vi "tsapp_configure_can_regs.vi"(8 "错误输入（无错误）":errorcluster, 10 "Cluster":T1, 11 "path":path) -> (0 "错误输出":errorcluster, 2 "Return Type":i32, 3 "path out":path)   [LabVIEW 2014]
doc: "Function Introduction :\nConfigure CAN sampling points and baud rate\nCall location :\nAfter connecting the hardware, it is necessary to create a diagnostic module\ninput parameter :\nAIdxChn: Channel Index\nABaud rate Kbps: baud rate\nASEG1: Arbitration Stage Phase Buffer Stage 1 ASEG2: Arbitration Stage Phase Buffer Stage 2 APrescaler: Arbitration Stage Frequency Division Coefficient\nASJW: BTL quantity\nAOnlyListen: Is it in listen only mode\nA120OhmConnected: Is the 120 Ω terminal resistor activated\nReturn value :\n0: Execution successful\nOther values: Failed"
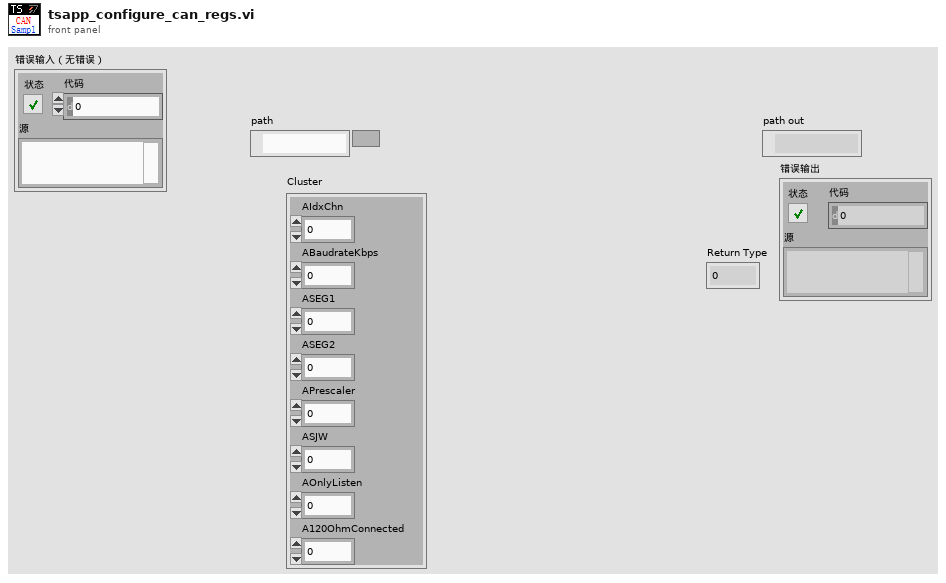
[diagram p1: front panel]
types:
  T1 = cluster{"AIdxChn":i32, "ABaudrateKbps":sgl, "ASEG1":i32, "ASEG2":i32, "APrescaler":i32, "ASJW":i32, "AOnlyListen":i32, "A120OhmConnected":i32}
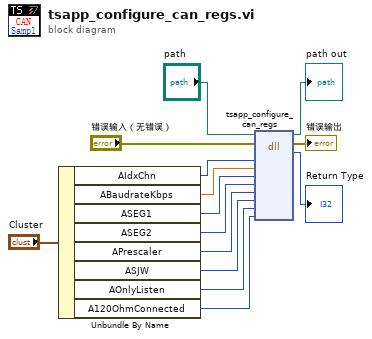
[diagram p0: block diagram]
diagram:
  n1 = Unbundle By Name("Cluster") -> ("AIdxChn"=w11:i32, "ABaudrateKbps"=w10:sgl, "ASEG1"=w8:i32, "ASEG2"=w9:i32, "APrescaler"=w7:i32, "ASJW"=w6:i32, "AOnlyListen"=w3:i32, "A120OhmConnected"=w4:i32)
  n2 = dll-call lib="C:/Users/XYY/Desktop/LabView Demo/TSCAN_LB2018_V1.3_20220301/Config/TSMaster.dll" fn="tsapp_configure_can_regs"(path in="path", error in="错误输入（无错误）", "AIdxChn"=w11, "ABaudrateKbps"=w10, "ASEG1"=w8, "ASEG2"=w9, "APrescaler"=w7, "ASJW"=w6, "AOnlyListen"=w3, "A120OhmConnected"=w4) -> (path out=→"path out":path, error out=→"错误输出":errorcluster, "返回类型"=→"Return Type":i32)  [unwired: 9 in]
